vi "[DAQmx] Close All.vi"() -> ()   [LabVIEW 2021]
panel:
  out "task in":refnum<k21>
  in  "Stop":bool
  in  "Close All session":bool
  out "DropDownList[]":string[](array[string])
  # "DAQmx Sessions"
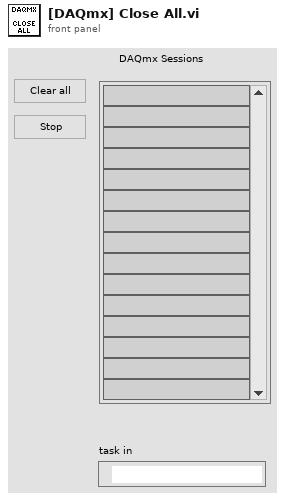
[diagram p1: front panel]
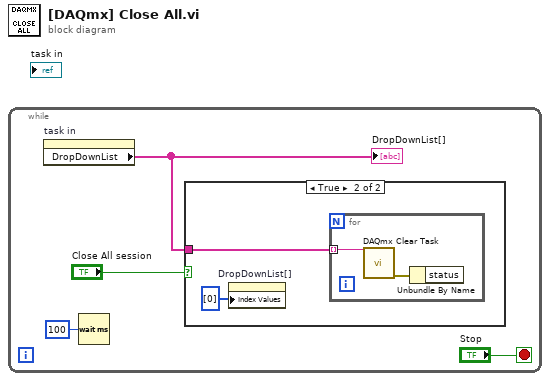
[diagram p0: block diagram]
diagram:
  n1 = while {
    stop <- "Stop" stop-if-true
    n2 = property on="task in" class="DAQmxName (strict)"() -> ("DropDownList"=w1:string[])  [unwired: 2 in, 2 out]
    "DropDownList[]" <- w1
    n3 = Wait (ms)(milliseconds to wait=u32 100) -> ()  [unwired: 1 out]
    n4 = case shown="True" "Close All session" {
      tunnel: w1 -> [_ w6]
      frame False {
      }
      frame True {
        n5 = property on="DropDownList[]" class="Arr (strict)"("Index Values"=u32[] [0]) -> ()  [unwired: 2 in, 2 out]
        n6 = for {
          tunnel: w6 -> [w8] mode=indexing
          n7 = call <vilib>:"DAQmx Clear Task.vi"("task in"=w8) -> ("error out"=w7:errorcluster)  [unwired: 14 in]
          n8 = Unbundle By Name(w7) -> ()  [unwired: 1 out]
        }
      }
    }
  }
